vi "dfd_CIC Bit Pruning.vi"(5 "cut?":bool, 7 "Bit to cut":i32, 11 "x":T1) -> (3 "y":T1)   [LabVIEW 2017, in "NI_DigFilter_FXP.lvlib"]
uses:
  <vilib>/addons/Digital Filter Design/NI_DigFilter_FXP.lvlib
  <vilib>/addons/Digital Filter Design/_Objects.llb/dfd_Integer I160.ctl
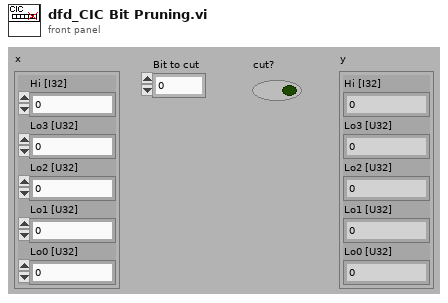
[diagram p1: front panel]
types:
  T1 = typedef "dfd_Integer I160.ctl" = cluster{"Hi [I32]":i32, "Lo3 [U32]":u32, "Lo2 [U32]":u32, "Lo1 [U32]":u32, "Lo0 [U32]":u32}
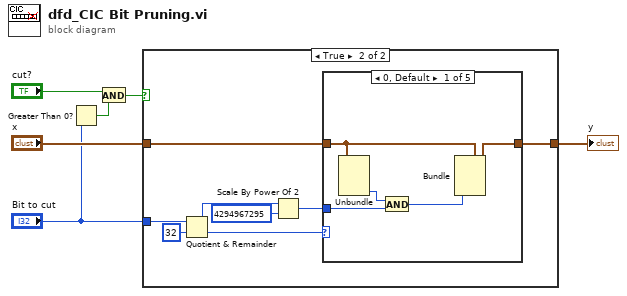
[diagram p0: block diagram]
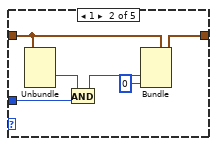
[diagram p3: hidden frame]
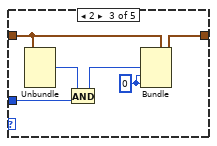
[diagram p4: hidden frame]
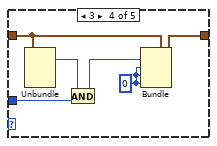
[diagram p5: hidden frame]
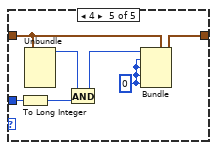
[diagram p6: hidden frame]
diagram:
  n1 = Greater Than 0?(x="Bit to cut") -> (x > 0?=w2:bool)
  n2 = And(x="cut?", y=w2) -> (x .and. y?=w3:bool)
  n3 = case shown="True" w3 {
    tunnel: "x" -> [w7 w10]
    tunnel: [w7 w9] -> w5
    tunnel: "Bit to cut" -> [_ w15]
    frame False {
    }
    frame True {
      n4 = Quotient & Remainder(x=w15, y=32) -> (x-y*floor(x/y)=w12:i32, floor(x/y)=w13:i32)
      n5 = Scale By Power Of 2(n=w12, x=u32 4294967295) -> (x*2^n=w8:u32)
      n6 = case shown="0, Default" w13 {
        tunnel: w10 -> [w20 w26 w32 w38 w45]
        tunnel: [w19 w25 w31 w37 w44] -> w9
        tunnel: w8 -> [w17 w24 w30 w36 w43]
        frame 0, Default {
          n7 = Unbundle(w20) -> ("Lo0 [U32]"=w18:u32)  [unwired: 4 out]
          n8 = And(x=w18, y=w17) -> (x .and. y?=w16:u32)
          n9 = Bundle(cluster=w20, "Lo0 [U32]"=w16) -> (w19:T1)  [unwired: 4 out]
        }
        frame 1 {
          n10 = Unbundle(w26) -> ("Lo1 [U32]"=w23:u32)  [unwired: 4 out]
          n11 = And(x=w23, y=w24) -> (x .and. y?=w22:u32)
          n12 = Bundle(cluster=w26, "Lo1 [U32]"=w22, "Lo0 [U32]"=u32 0) -> (w25:T1)  [unwired: 3 out]
        }
        frame 2 {
          w27 = u32 0 ("Lo0 [U32]")
          n13 = Unbundle(w32) -> ("Lo2 [U32]"=w29:u32)  [unwired: 4 out]
          n14 = And(x=w29, y=w30) -> (x .and. y?=w28:u32)
          n15 = Bundle(cluster=w32, "Lo2 [U32]"=w28, "Lo1 [U32]"=w27, "Lo0 [U32]"=w27) -> (w31:T1)  [unwired: 2 out]
        }
        frame 3 {
          w33 = u32 0 ("Lo0 [U32]")
          n16 = Unbundle(w38) -> ("Lo3 [U32]"=w35:u32)  [unwired: 4 out]
          n17 = And(x=w35, y=w36) -> (x .and. y?=w34:u32)
          n18 = Bundle(cluster=w38, "Lo3 [U32]"=w34, "Lo2 [U32]"=w33, "Lo1 [U32]"=w33, "Lo0 [U32]"=w33) -> (w37:T1)  [unwired: 1 out]
        }
        frame 4 {
          w40 = u32 0 ("Lo0 [U32]")
          n19 = To Long Integer(number=w43) -> (32bit integer=w39:i32)
          n20 = Unbundle(w45) -> ("Hi [I32]"=w42:i32)  [unwired: 4 out]
          n21 = And(x=w42, y=w39) -> (x .and. y?=w41:i32)
          n22 = Bundle(cluster=w45, "Hi [I32]"=w41, "Lo3 [U32]"=w40, "Lo2 [U32]"=w40, "Lo1 [U32]"=w40, "Lo0 [U32]"=w40) -> (w44:T1)
        }
      }
    }
  }
  "y" <- w5
